vi "test Add Script Deploy.vi"(8 "error in":errorcluster, 11 "TestCase in":refnum<class "Examples.lvclass">) -> (0 "error out":errorcluster, 3 "TestCase out":refnum<class "Examples.lvclass">)   [LabVIEW 2020, in "Examples.lvclass"]
uses:
  Examples.lvclass
  C:/Git/niveristand-custom-device-testing-tools/VeriStandTestCase/VeriStandTestCase.lvclass
  Shared/Device Parameters.ctl
  Shared/Initialization Method.ctl
  Shared/Direction.ctl
  Shared/SDI.ctl
  Shared/Transfer Type.ctl
  Shared/Parameter Definition.ctl
  Encoding and Decoding/Encoding.ctl
  Examples.lvclass/Examples.ctl
  7f6914e5-79d7-41a5-a6cd-be6651e4326d.vi
  <vilib>/addons/_JKI Toolkits/VI Tester/TestCase.llb/TestCase.lvclass
  Scripting/Ballard/Ballard ARINC 429 Scripting.lvlib
  niveristand-custom-device-testing-tools/VeriStandTestUtilities/VeriStandTestUtilities.lvlib
  Encoding and Decoding/Encoding and Decoding.lvlib
  C:/Program Files (x86)/National Instruments/LabVIEW 2020/vi.lib/addons/_JKI Toolkits/VI Tester/TestCase.llb/TestCase.lvclass
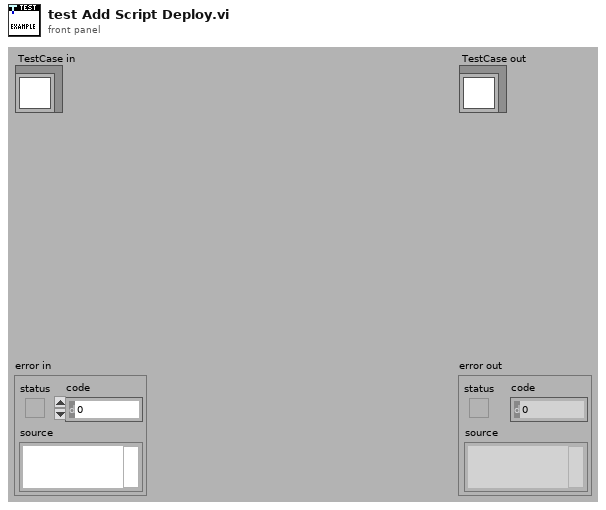
[diagram p1: front panel]
types:
  T1 = typedef "Direction.ctl" = enum16{"Rx", "Tx"}
  T2 = typedef "Device Parameters.ctl" = cluster{"initialization method":T3, "card number":i32, "PXI slot number":i32, "core number":i32}
  T3 = typedef "Initialization Method.ctl" = enum16{"PXI Slot Number", "Card Number"}
  T4 = typedef "Parameter Definition.ctl" = cluster{"start index":i32, "size":i32, "encoding":T5, "signed":bool, "scale multiplier":dbl, "scale offset":dbl}
  T5 = typedef "Encoding and Decoding.lvlib/Encoding.ctl" = enum16{"BNR", "BCD", "Discrete"}
  T6 = typedef "Transfer Type.ctl" = enum16{"Scheduled", "Acyclic", "Block", "Strobe"}
  T7 = typedef "SDI.ctl" = i32
  T8 = cluster{"name":string, "unit":string, "default value":dbl}[]
  T9 = typedef "Custom Device API.lvlib/Custom Device Item Ref.ctl" = u64
  T10 = typedef "NI_VS Workspace ExecutionAPI.lvlib/WorkspaceAPI.ctl" = refnum<k24>
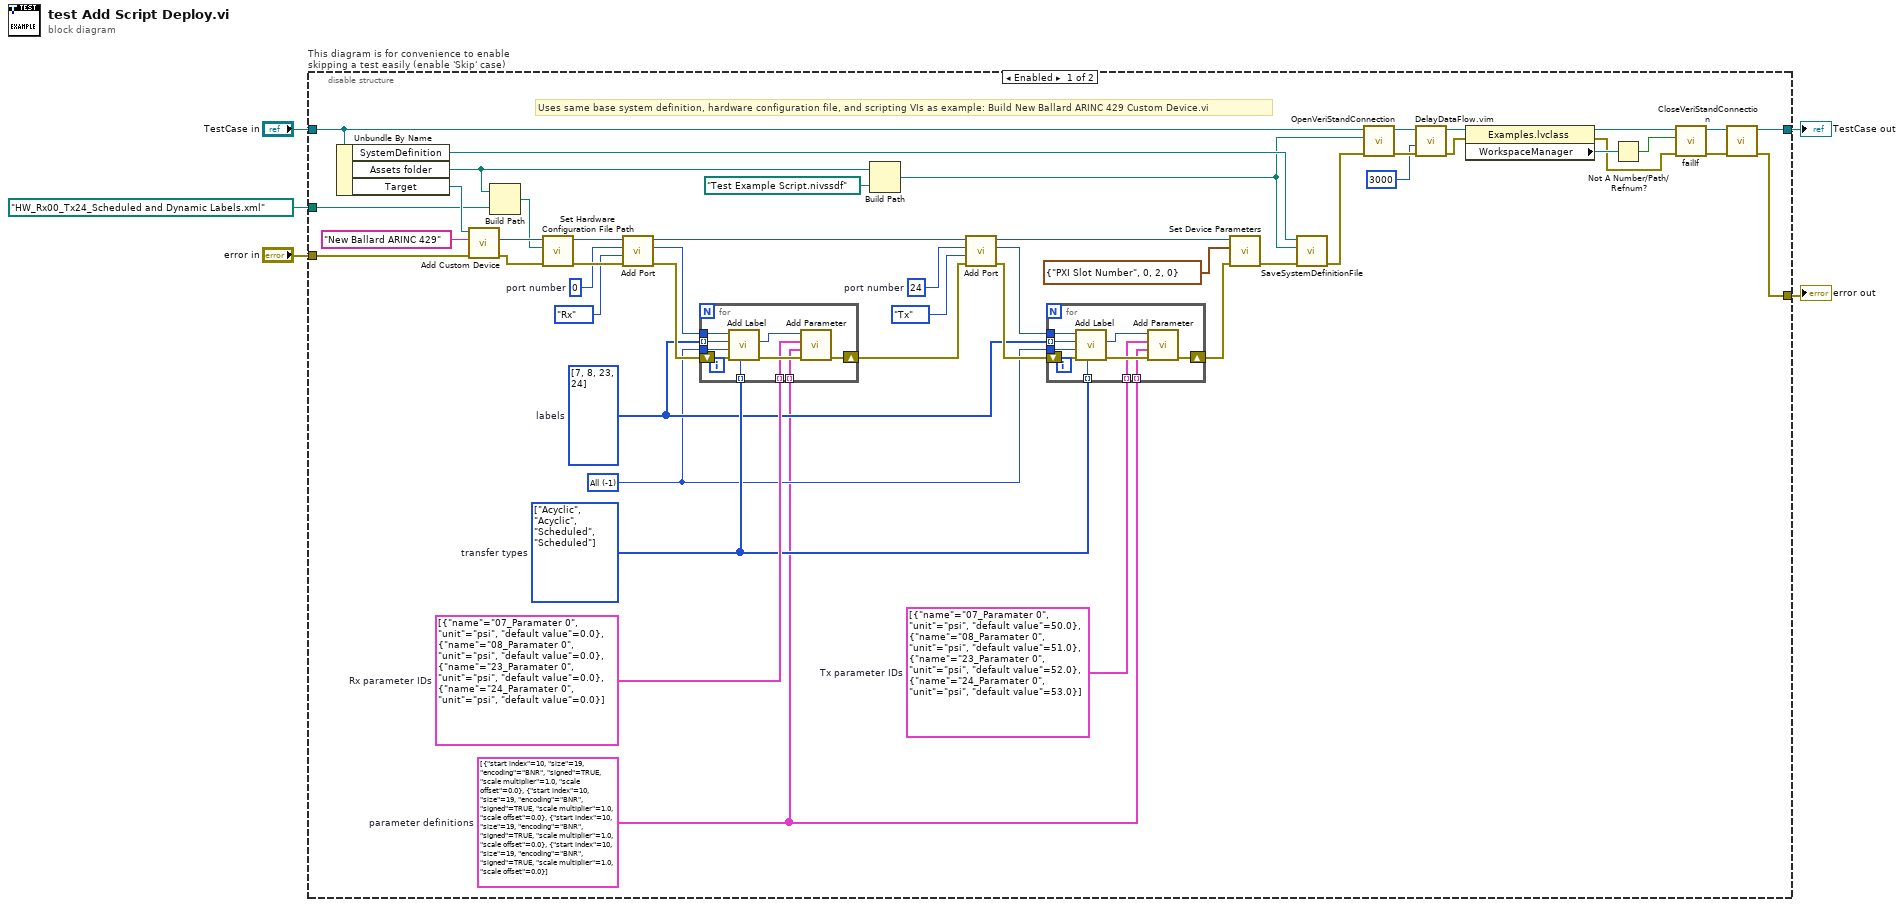
[diagram p0: block diagram]
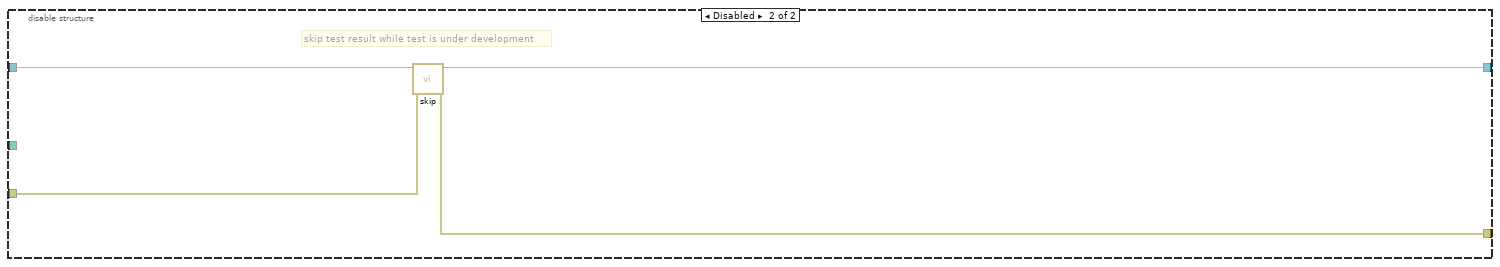
[diagram p2: hidden frame]
diagram:
  n1 = disable-structure "This diagram is for convenience to enable skipping a test easily (enable 'Skip' case)" shown="Enabled" {
    disable-tunnel: "TestCase in" -> [w35 w76]
    disable-tunnel: [w36 w74] -> w2
    disable-tunnel: [w37 w75] -> w4
    disable-tunnel: "error in" -> [w34 w73]
    disable-tunnel: path "HW_Rx00_Tx24_Scheduled and Dynamic Labels.xml" ("name or relative path") -> [w31 _]
    frame Enabled {
      w7 = T4[] [{"start index"=10, "size"=19, "encoding"=enum."BNR", "signed"=TRUE, "scale multiplier"=1.0, "scale offset"=0.0}, {"start index"=10, "size"=19, "encoding"=enum."BNR", "signed"=TRUE, "scale multiplier"=1.0, "scale offset"=0.0}, {"start index"=10, "size"=19, "encoding"=enum."BNR", "signed"=TRUE, "scale multiplier"=1.0, "scale offset"=0.0}, {"start index"=10, "size"=19, "encoding"=enum."BNR", "signed"=TRUE, "scale multiplier"=1.0, "scale offset"=0.0}]  # parameter definitions
      w11 = T6[] [enum."Acyclic", enum."Acyclic", enum."Scheduled", enum."Scheduled"] items=["Scheduled", "Acyclic", "Block", "Strobe"]  # transfer types
      w9 = T7 -1 items=["All"=-1, "0 (b00)"=0, "1 (b01)"=1, "2 (b10)"=2, "3 (b11)"=3] ("SDI value")
      w8 = T8 [{"name"="07_Paramater 0", "unit"="psi", "default value"=50.0}, {"name"="08_Paramater 0", "unit"="psi", "default value"=51.0}, {"name"="23_Paramater 0", "unit"="psi", "default value"=52.0}, {"name"="24_Paramater 0", "unit"="psi", "default value"=53.0}]  # Tx parameter IDs
      w15 = T8 [{"name"="07_Paramater 0", "unit"="psi", "default value"=0.0}, {"name"="08_Paramater 0", "unit"="psi", "default value"=0.0}, {"name"="23_Paramater 0", "unit"="psi", "default value"=0.0}, {"name"="24_Paramater 0", "unit"="psi", "default value"=0.0}]  # Rx parameter IDs
      w19 = u16 24  # port number
      w10 = u32[] [7, 8, 23, 24]  # labels
      w21 = u16 0  # port number
      # "Uses same base system definition, hardware configuration file, and scripting VIs as example: Build New Ballard ARINC 429 Custom Device.vi"
      n2 = Unbundle By Name(w35) -> ("SystemDefinition"=w32:refnum<k24>, "Assets folder"=w30:path, "Target"=w52:refnum<k24>)
      n3 = call "Add Custom Device.vi"("error in"=w34, "name"="New Ballard ARINC 429", "target in"=w52) -> ("error out"=w50:errorcluster, "Ballard ARINC 429 ref out"=w51:T9)  [unwired: 6 in, 1 out]
      n4 = Build Path(base path=w30, name or relative path=w31) -> (appended path=w49:path)
      n5 = call "Set Hardware Configuration File Path.vi"("error in"=w50, "path"=w49, "custom device ref"=w51) -> ("error out"=w22:errorcluster, "custom device ref out"=w24:T9)  [unwired: 7 in]
      n6 = call "Add Port.vi"("error in"=w22, "direction"=Direction."Rx", "port number"=w21, "custom device ref"=w24) -> ("error out"=w16:errorcluster, "port ref out"=w17:T9, "custom device ref out"=w25:T9)  [unwired: 5 in]
      n7 = for {
        tunnel: w17 -> [w62]
        shift-right: [w53] -> w13
        shift-left: w16 -> [w61]
        tunnel: w10 -> [w60] mode=indexing
        tunnel: w11 -> [w57] mode=indexing
        tunnel: w9 -> [w56]
        tunnel: w15 -> [w55] mode=indexing
        tunnel: w7 -> [w54] mode=indexing
        n8 = call "Add Label.vi"("transfer type"=w57, "error in"=w61, "SDI value"=w56, "label value"=w60, "port ref"=w62) -> ("error out"=w58:errorcluster, "label ref"=w59:T9)  [unwired: 4 in, 1 out]
        n9 = call "Add Parameter.vi"("error in"=w58, "parameter definition"=w54, "parameter"=w55, "label ref"=w59) -> ("error out"=w53:errorcluster)  [unwired: 5 in, 2 out]
      }
      n10 = Build Path(base path=w30, name or relative path=path "Test Example Script.nivssdf") -> (appended path=w28:path)
      n11 = call "Add Port.vi"("error in"=w13, "direction"=Direction."Tx", "port number"=w19, "custom device ref"=w25) -> ("error out"=w12:errorcluster, "port ref out"=w14:T9, "custom device ref out"=w23:T9)  [unwired: 5 in]
      n12 = for {
        tunnel: w14 -> [w72]
        shift-right: [w63] -> w6
        shift-left: w12 -> [w71]
        tunnel: w10 -> [w70] mode=indexing
        tunnel: w11 -> [w67] mode=indexing
        tunnel: w9 -> [w66]
        tunnel: w8 -> [w65] mode=indexing
        tunnel: w7 -> [w64] mode=indexing
        n13 = call "Add Label.vi"("transfer type"=w67, "error in"=w71, "SDI value"=w66, "label value"=w70, "port ref"=w72) -> ("error out"=w68:errorcluster, "label ref"=w69:T9)  [unwired: 4 in, 1 out]
        n14 = call "Add Parameter.vi"("error in"=w68, "parameter definition"=w64, "parameter"=w65, "label ref"=w69) -> ("error out"=w63:errorcluster)  [unwired: 5 in, 2 out]
      }
      n15 = call "Set Device Parameters.vi"("error in"=w6, "device parameters"=T2 {"initialization method"=enum."PXI Slot Number", "card number"=0, "PXI slot number"=2, "core number"=0}, "Ballard ARINC 429 custom device in"=w23) -> ("error out"=w27:errorcluster)  [unwired: 7 in, 1 out]
      n16 = call "SaveSystemDefinitionFile.vi"("error in (no error)"=w27, "System Definition File in"=w28, "System Definition Reference in"=w32) -> ("error out"=w38:errorcluster)  [unwired: 7 in, 1 out]
      n17 = call-dynamic "OpenVeriStandConnection.vi"("error in (no error)"=w38, "System Definition File"=w28, "VeriStand Test Case in"=w35) -> ("error out"=w41:errorcluster, "VeriStand Test Case out"=w40:refnum<class "Examples.lvclass">)  [unwired: 6 in, 1 out]
      n18 = call "DelayDataFlow.vim"("value in"=w41, "milliseconds to wait"=u32 3000) -> ("value out"=w48:errorcluster)  [unwired: 2 in, 1 out]
      n19 = property class="Examples.lvclass"(reference=w40, error in=w48) -> (reference out=w47:refnum<class "Examples.lvclass">, error out=w42:errorcluster, "WorkspaceManager"=w44:T10)
      n20 = Not A Number/Path/Refnum?(number/path/refnum=w44) -> (NaN/Path/Refnum?=w43:bool)
      n21 = call-dynamic "failIf.vi"("error in (no error)"=w42, "fail"=w43, "TestCase in"=w47) -> ("error out"=w45:errorcluster, "TestCase out"=w46:refnum<class "Examples.lvclass">)  [unwired: 7 in]
      n22 = call-dynamic "CloseVeriStandConnection.vi"("error in (no error)"=w45, "VeriStand Test Case in"=w46) -> ("error out"=w37:errorcluster, "VeriStand Test Case out"=w36:refnum<class "Examples.lvclass">)  [unwired: 8 in]
    }
    frame Disabled {
      # "skip test result while test is under development"
      n23 = call <vilib>:"skip.vi"("error in (no error)"=w73, "TestCase in"=w76) -> ("error out"=w75:errorcluster, "TestCase out"=w74:refnum<class "Examples.lvclass">)  [unwired: 8 in]
    }
  }
  "error out" <- w4
  "TestCase out" <- w2
